vi "Player Info.vi"(11 "Sentinel in":refnum<class "Sentinel.lvclass">) -> (1 "Victory Speech":string, 2 "Name":string, 3 "Sentinel out":refnum<class "Sentinel.lvclass">)   [LabVIEW 2015, in "Sentinel.lvclass"]
uses:
  Sentinel.lvclass
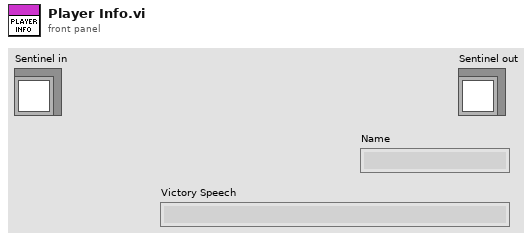
[diagram p1: front panel]
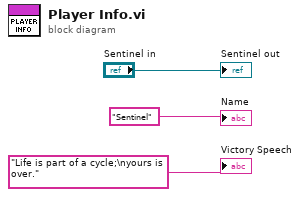
[diagram p0: block diagram]
diagram:
  "Sentinel out" <- "Sentinel in"
  "Name" <- "Sentinel"
  "Victory Speech" <- "Life is part of a cycle;\nyours is over."
